vi "CheckTestEngineModel.vi"(11 "Modle":string) -> (3 "Pattern":string)   [LabVIEW 2019, in "TestBench.lvlib" / "TestBench.lvclass"]
uses:
  TestBench.lvclass
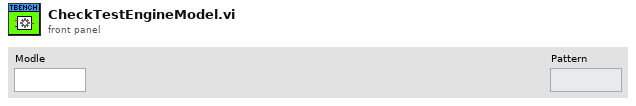
[diagram p1: front panel]
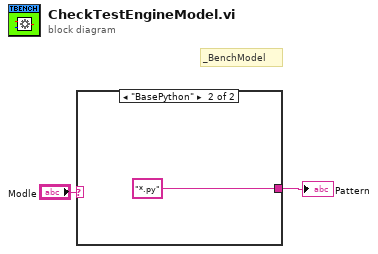
[diagram p0: block diagram]
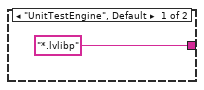
[diagram p2: hidden frame]
diagram:
  # "_BenchModel"
  n1 = case shown="\"BasePython\"" "Modle" {
    tunnel: ["*.lvlibp" ("regular expression") "*.py" ("regular expression")] -> w1
    frame "UnitTestEngine", Default {
    }
    frame "BasePython" {
    }
  }
  "Pattern" <- w1
